vi "IO_PumpCmdMsg.vi"(6 "Enable":bool=TRUE, 8 "Drain Signal":bool, 9 "FIll Signal":bool, 10 "Pump Speed":enum16{"FAST", "SLOW", "CREEP", "STOP"}(ring)=enum."STOP", 11 "Cmd IN":u32=56) -> (0 "Pump State Out":enum16{"INIT", "IDLE", "STOP", "FILL", "DRAIN"}(ring)=enum."FILL", 1 "Msg Active":bool, 2 "Message":string[](array[string])=["dout 80"], 3 "Cmd Out":u32=80)   [LabVIEW 2024]
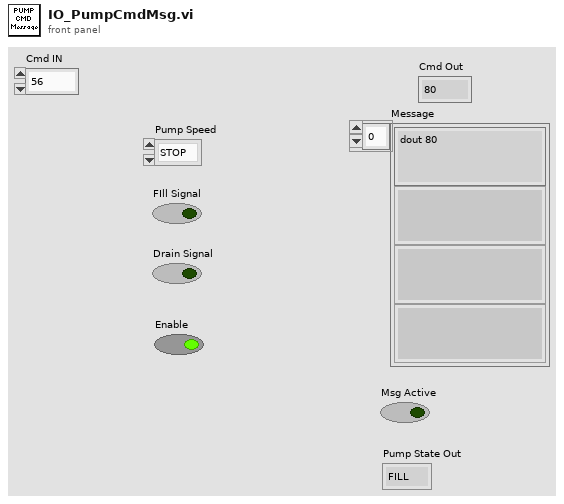
[diagram p1: front panel]
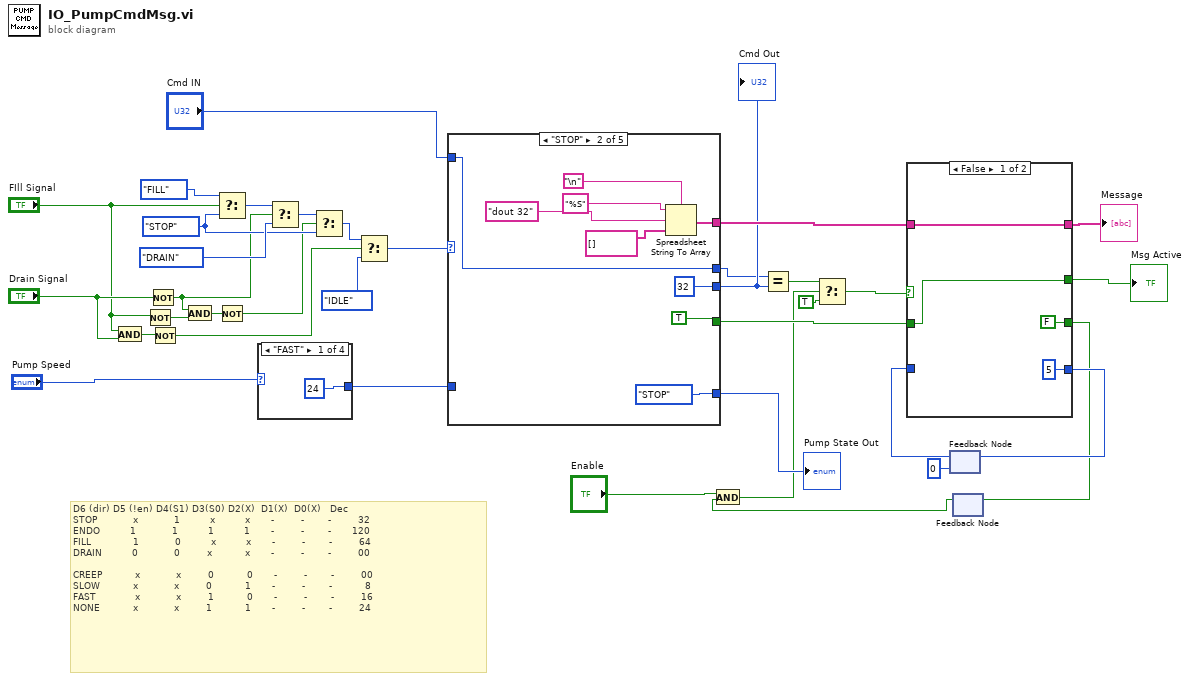
[diagram p0: block diagram]
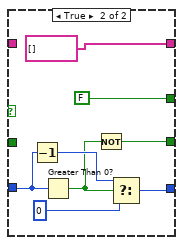
[diagram p2: hidden frame]
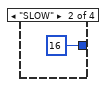
[diagram p3: hidden frame]
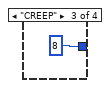
[diagram p4: hidden frame]
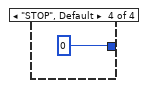
[diagram p5: hidden frame]
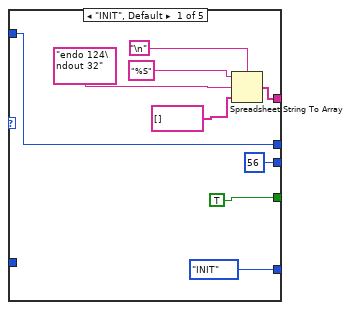
[diagram p6: hidden frame]
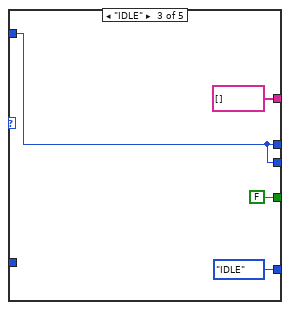
[diagram p7: hidden frame]
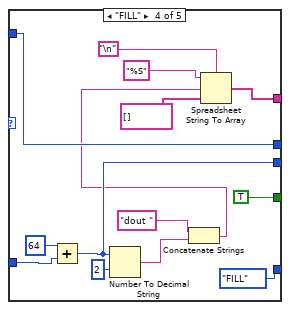
[diagram p8: hidden frame]
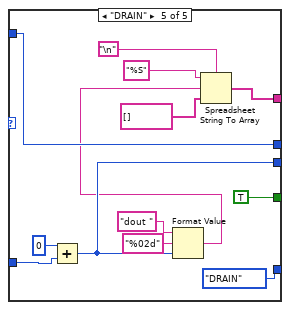
[diagram p9: hidden frame]
diagram:
  w32 = enum16{"INIT", "IDLE", "STOP", "FILL", "DRAIN"}."STOP" ("State")
  # "D6 (dir) D5 (!en) D4(S1) D3(S0) D2(X)  D1(X)  D0(X)   Dec\nSTOP            x            1          x          x       -         -        -         32\nENDO          1            1          1          1       -         -        -       120\nFILL              1            0          x          x       -         -        -         64\nDRAIN          0            0         x           x       -         -        -         00\n\nCREEP           x            x         0           0       -         -        -         00    \nSLOW           x            x         0           1       -         -        -           8\nFAST             x            x         1           0       -         -        -         16\nNONE           x            x         1           1       -         -        -         24"
  n1 = And(x="FIll Signal", y="Drain Signal") -> (x .and. y?=w15:bool)
  n2 = Not(x="FIll Signal") -> (.not. x?=w21:bool)
  n3 = Not(x="Drain Signal") -> (.not. x?=w20:bool)
  n4 = Not(x=w15) -> (.not. x?=w14:bool)
  n5 = And(x=w20, y=w21) -> (x .and. y?=w19:bool)
  n6 = Select(t=enum16{"INIT", "IDLE", "STOP", "FILL", "DRAIN"}."FILL" ("State"), s="FIll Signal", f=w32) -> (s? t:f=w35:enum16{"INIT", "IDLE", "STOP", "FILL", "DRAIN"})
  n7 = Not(x=w19) -> (.not. x?=w18:bool)
  n8 = case shown="\"FAST\"" "Pump Speed" {
    tunnel: [u32 24 ("number") u32 16 ("number") u32 8 ("number") u32 0 ("number")] -> w30
    frame "FAST" {
    }
    frame "SLOW" {
    }
    frame "CREEP" {
    }
    frame "STOP", Default {
    }
  }
  n9 = Select(t=w35, s=w20, f=enum16{"INIT", "IDLE", "STOP", "FILL", "DRAIN"}."DRAIN" ("State")) -> (s? t:f=w33:enum16{"INIT", "IDLE", "STOP", "FILL", "DRAIN"})
  n10 = Select(t=w33, s=w18, f=w32) -> (s? t:f=w17:enum16{"INIT", "IDLE", "STOP", "FILL", "DRAIN"})
  n11 = Select(t=w17, s=w14, f=enum16{"INIT", "IDLE", "STOP", "FILL", "DRAIN"}."IDLE") -> (s? t:f=w12:enum16{"INIT", "IDLE", "STOP", "FILL", "DRAIN"})
  n12 = case shown="\"STOP\"" w12 {
    tunnel: [w46 w55 string[] [] w64 w82] -> w24
    tunnel: [TRUE TRUE FALSE TRUE TRUE] -> w25
    tunnel: [enum16{"INIT", "IDLE", "STOP", "FILL", "DRAIN"}."INIT" ("State") enum16{"INIT", "IDLE", "STOP", "FILL", "DRAIN"}."STOP" ("State") enum16{"INIT", "IDLE", "STOP", "FILL", "DRAIN"}."IDLE" ("State") enum16{"INIT", "IDLE", "STOP", "FILL", "DRAIN"}."FILL" ("State") enum16{"INIT", "IDLE", "STOP", "FILL", "DRAIN"}."DRAIN" ("State")] -> w26
    tunnel: w30 -> [_ _ _ w71 w87]
    tunnel: [u32 56 u32 32 w61 w69 w80] -> w23
    tunnel: "Cmd IN" -> [w41 w50 w61 w68 w85]
    tunnel: [w41 w50 w61 w68 w85] -> w13
    frame "INIT", Default {
      n13 = Spreadsheet String To Array(delimiter (Tab)="\n", format string="%S", spreadsheet string="endo 124\ndout 32" ("Command List"), array type (2D Dbl)=string[] []) -> (array=w46:string[])
    }
    frame "STOP" {
      n14 = Spreadsheet String To Array(delimiter (Tab)="\n", format string="%S", spreadsheet string="dout 32", array type (2D Dbl)=string[] []) -> (array=w55:string[])
    }
    frame "IDLE" {
    }
    frame "FILL" {
      n15 = Add(x=u32 64 ("number"), y=w71) -> (x+y=w69:u32)
      n16 = Number To Decimal String(number=w69, width (-)=i16 2) -> (decimal integer string=w72:string)
      n17 = Concatenate Strings("dout " ("string"), w72) -> (w63:string)
      n18 = Spreadsheet String To Array(delimiter (Tab)="\n", format string="%S", spreadsheet string=w63, array type (2D Dbl)=string[] []) -> (array=w64:string[])
    }
    frame "DRAIN" {
      n19 = Add(x=u32 0 ("number"), y=w87) -> (x+y=w80:u32)
      n20 = Format Value(string ("")="dout " ("string"), format string="%02d", value (0)=w80) -> (output string=w79:string)
      n21 = Spreadsheet String To Array(delimiter (Tab)="\n", format string="%S", spreadsheet string=w79, array type (2D Dbl)=string[] []) -> (array=w82:string[])
    }
  }
  "Pump State Out" <- w26
  "Cmd Out" <- w23
  n22 = Equal?(x=w13, y=w23) -> (x = y?=w10:bool)
  n23 = feedback #1(0 ("f")) -> (w6:i32)
  n24 = feedback #2() -> (w2:bool)  [unwired: 1 in]
  n25 = And(x="Enable", y=w2) -> (x .and. y?=w5:bool)
  n26 = Select(t=w10, s=w5, f=TRUE) -> (s? t:f=w8:bool)
  n27 = case shown="False" w8 {
    tunnel: [w93 string[] []] -> w28
    tunnel: [w92 FALSE] -> w27
    tunnel: w25 -> [w92 _]
    tunnel: w24 -> [w93 _]
    tunnel: [5 ("f") w96] -> w7
    tunnel: w6 -> [_ w94]
    tunnel: [FALSE w95] -> w3
    frame False {
    }
    frame True {
      n28 = Decrement(x=w94) -> (x-1=w99:i32)
      n29 = Greater Than 0?(x=w94) -> (x > 0?=w97:bool)
      n30 = Not(x=w97) -> (.not. x?=w95:bool)
      n31 = Select(t=w99, s=w97, f=0) -> (s? t:f=w96:i32)
    }
  }
  "Message" <- w28
  "Msg Active" <- w27
  n32 = feedback-in #1(w7) -> ()
  n33 = feedback-in #2(w3) -> ()
